vi "CLSUIP_Populate Parent Interface Tree Based on Names.vi"(6 "Hide Missing (F)":bool, 7 "Parent Interface IDs and References":T1[](array[typedef]), 8 "error in (no error)":errorcluster, 9 "Class":refnum<vi>, 10 "Parent Class":refnum<vi>, 11 "Parent Interface Tree":refnum<vi>) -> (0 "error out":errorcluster, 2 "Show Remove Missing?":bool, 3 "Show Legend?":bool)   [LabVIEW 2021]
uses:
  <resource>/Framework/Providers/LVClassLibrary/CLSUIP_ItemID Reference Pair.ctl
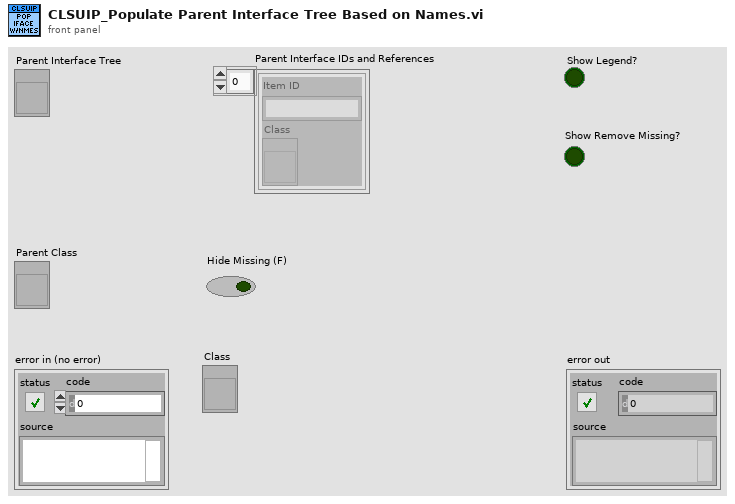
[diagram p1: front panel]
types:
  T1 = typedef "CLSUIP_ItemID Reference Pair.ctl" = cluster{"Item ID":string, "Class":refnum<vi>}
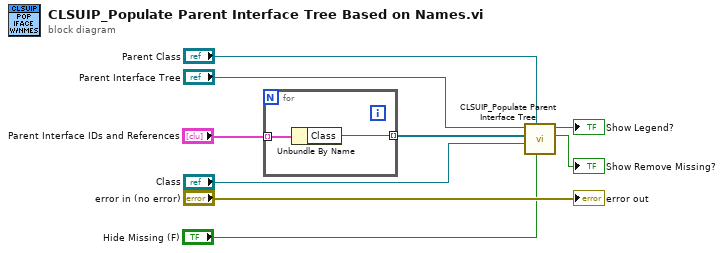
[diagram p0: block diagram]
diagram:
  n1 = for {
    tunnel: "Parent Interface IDs and References" -> [w11] mode=indexing
    tunnel: [w10] -> w4 mode=indexing
    n2 = Unbundle By Name(w11) -> ("Class"=w10:refnum<vi>)
  }
  n3 = call <resource>:"CLSUIP_Populate Parent Interface Tree.vi"("Hide Missing (F)"="Hide Missing (F)", "Parent Class"="Parent Class", "Class"="Class", "Parent Interfaces"=w4, "Tree"="Parent Interface Tree") -> ("Show Remove Missing?"=→"Show Remove Missing?":bool, "Show Legend?"=→"Show Legend?":bool)  [unwired: 5 in]
  "error out" <- "error in (no error)"
